vi "Acceleration-Set.vi"(11 "計算設置":cluster{"總位移量":dbl, "最高速":dbl, "加速度":dbl}) -> (3 "輸出結果":T1)   [LabVIEW 2019]
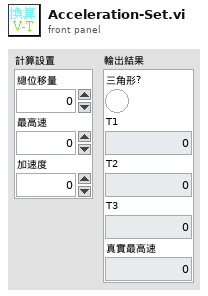
[diagram p1: front panel]
types:
  T1 = cluster{"三角形?":bool, "T1":dbl, "T2":dbl, "T3":dbl, "真實最高速":dbl}
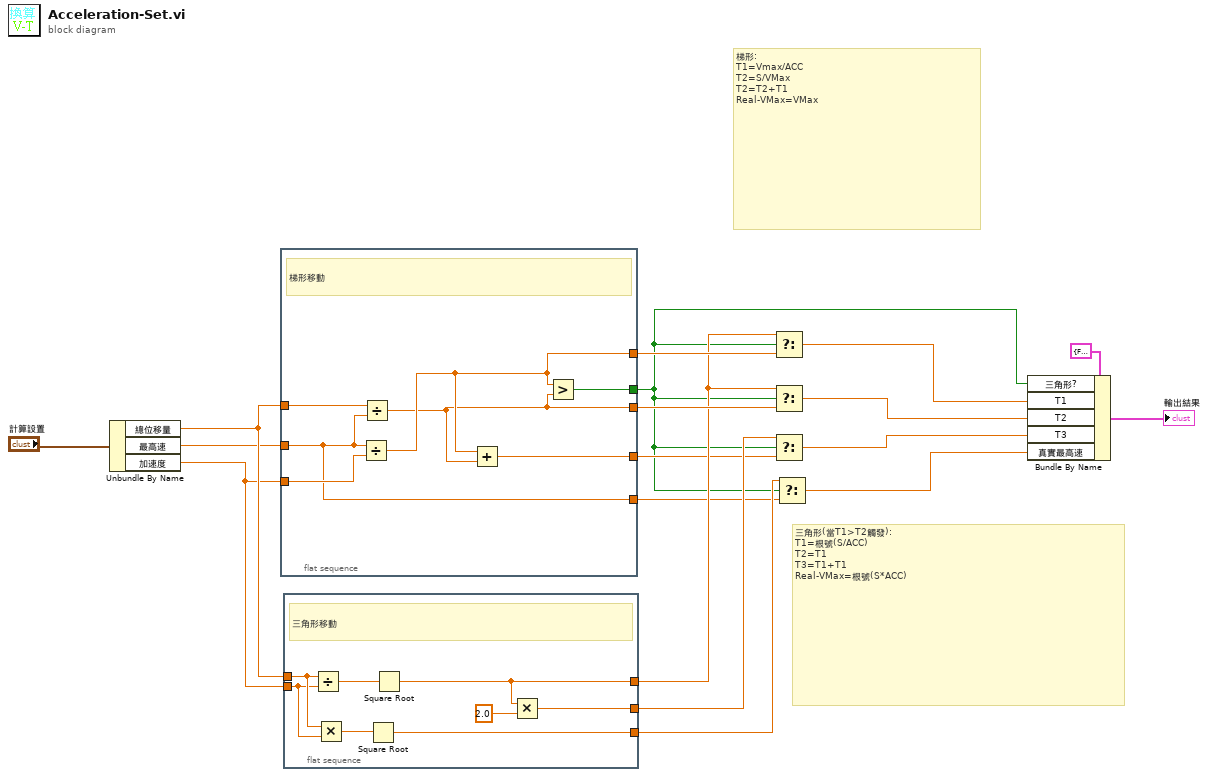
[diagram p0: block diagram]
diagram:
  # "三角形(當T1>T2觸發):\nT1=根號(S/ACC)\nT2=T1\nT3=T1+T1\nReal-VMax=根號(S*ACC)"
  # "梯形:\nT1=Vmax/ACC\nT2=S/VMax\nT2=T2+T1\nReal-VMax=VMax"
  n1 = Unbundle By Name("計算設置") -> ("總位移量"=w6:dbl, "最高速"=w5:dbl, "加速度"=w4:dbl)
  n2 = flat-sequence {
    tunnel: w4 -> [w25]
    tunnel: w5 -> [w19]
    tunnel: w6 -> [w24]
    tunnel: [w23] -> w11
    tunnel: [w22] -> w18
    tunnel: [w21] -> w17
    tunnel: [w20] -> w14
    tunnel: [w19] -> w12
    frame #0 {
      # "梯形移動"
      n3 = Divide(x=w19, y=w25) -> (x/y=w22:dbl)
      n4 = Divide(x=w24, y=w19) -> (x/y=w21:dbl)
      n5 = Add(x=w22, y=w21) -> (x+y=w20:dbl)
      n6 = Greater?(x=w22, y=w21) -> (0:w23:bool)
    }
  }
  n7 = flat-sequence {
    tunnel: w6 -> [w29]
    tunnel: w4 -> [w28]
    tunnel: [w32] -> w16
    tunnel: [w30] -> w15
    tunnel: [w26] -> w13
    frame #0 {
      # "三角形移動"
      n8 = Divide(x=w29, y=w28) -> (x/y=w33:dbl)
      n9 = Multiply(x=w29, y=w28) -> (x*y=w27:dbl)
      n10 = Square Root(x=w27) -> (sqrt(x)=w26:dbl)
      n11 = Square Root(x=w33) -> (sqrt(x)=w32:dbl)
      n12 = Multiply(x=w32, y=2.0) -> (x*y=w30:dbl)
    }
  }
  n13 = Select(t=w16, s=w11, f=w18) -> (s? t:f=w10:dbl)
  n14 = Select(t=w16, s=w11, f=w17) -> (s? t:f=w9:dbl)
  n15 = Select(t=w15, s=w11, f=w14) -> (s? t:f=w8:dbl)
  n16 = Select(t=w13, s=w11, f=w12) -> (s? t:f=w7:dbl)
  n17 = Bundle By Name(cluster=T1 {"三角形?"=FALSE, "T1"=1.4142135623730951, "T2"=1.4142135623730951, "T3"=2.8284271247461903, "真實最高速"=70.71067811865476} ("輸出數值"), "三角形?"=w11, "T1"=w10, "T2"=w9, "T3"=w8, "真實最高速"=w7) -> (→"輸出結果":T1)
